vi "系统设置.vi"() -> ()   [LabVIEW 2016]
uses:
  <vilib>/Utility/miscctls.llb/LVPointTypeDef.ctl
  <vilib>/ptbypt/NI_PtbyPt.lvlib
  <vilib>/Utility/config.llb/NI_LVConfig.lvlib
  PLC/PLC.lvlib
panel:
  in  "模块启用配置":bool
  in  "短信报警设置":bool
  in  "首页显示设置":bool
  in  "跨度核查":bool
  in  "空白核查":bool
  out "选项卡控件":enum32{"自由设定", "国标协议", "流量设定"}(tab)
  in  "24H周期设置":bool[](xcontrol)
  in  "运行间隔":i16=4 min=1 max=24
  in  "流量阈值":dbl=4.0 min=1.0 max=24.0
  in  "时间阈值":u16=4 min=1 max=24
  in  "周期设置":enum16{"自由设定", "国标协议", "流量设定"}(ring)
  out "x = y?":bool
  in  "质控启动日期":string(combo)="关闭"
  in  "跨度核查时间":u16(ring)=6 items=["00H", "01H", "02H", "03H", "04H", "05H", "06H", "07H", "08H", "09H", "10H", "11H", "12H", "13H", "14H", "15H", "16H", "17H", "18H", "19H", "20H", "21H", "22H", "23H", "关闭"]
  in  "空白核查时间":u16(ring)=2 items=["00H", "01H", "02H", "03H", "04H", "05H", "06H", "07H", "08H", "09H", "10H", "11H", "12H", "13H", "14H", "15H", "16H", "17H", "18H", "19H", "20H", "21H", "22H", "23H", "关闭"]
  in  "CODCr":bool
  in  "总磷总氮":bool
  in  "氨氮":bool
  in  "CODmn":bool
  in  "多参数":bool
  in  "输入密码":dbl
  in  "布尔":bool
  in  "副屏显示设置":bool
  in  "开机启动":bool caption="氨氮禁用"
  in  "运行模式":enum16{"维护模式", "常规模式", "应急模式", "质控模式"}(ring)
  # "注：周期设置分为自由设定和国标协议两种。\n1：选择自由设定情况下：运行间隔将不可选用并变灰色，周期设置可自由手动勾选\n2：选择国标协议情况下：周期时间将由运行间隔选择的时间决定，下方周期设置被禁用并无法手动勾选。\n3：选择流量设定情况下：瞬时流量连续超过流量阈值到达时间阈值设定值，仪器将自动开启测量。"
  # "自动运行启动参数"
  # "质控频次："
  # "空白核查时间："
  # "跨度核查时间："
  # "启动周期设置"
  # "m3/S"
  # "秒"
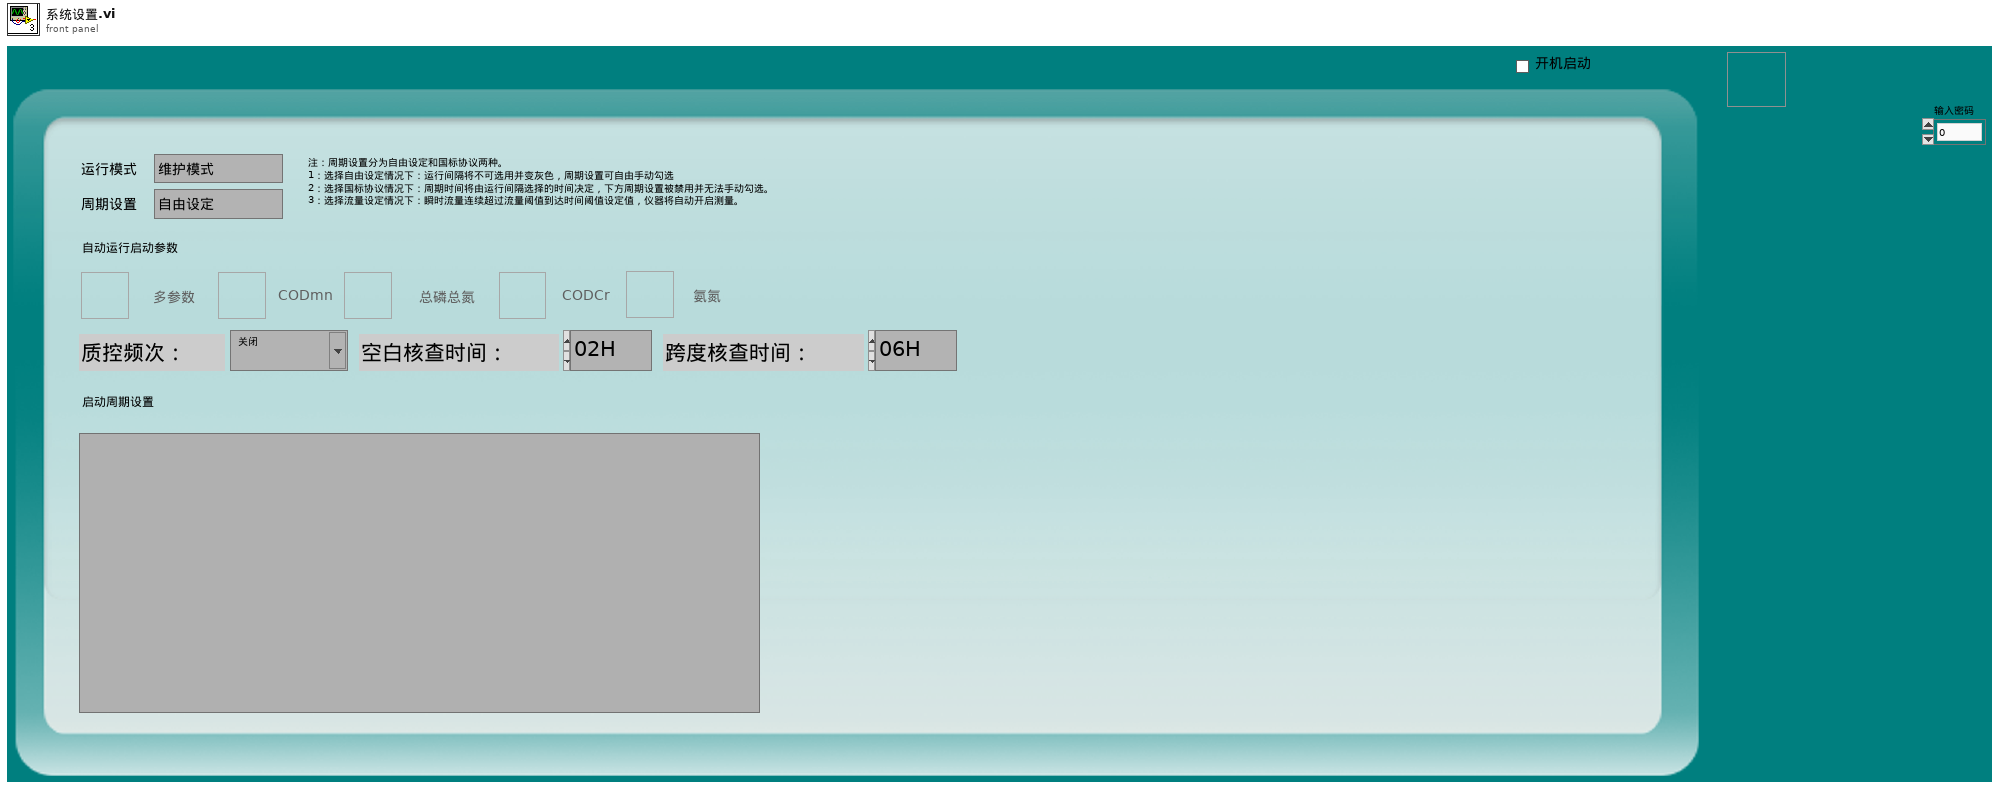
[diagram p1: front panel]
types:
  T1 = typedef "NI_LVConfig.lvlib/Config Data RefNum.ctl" = refnum<k1>
  T2 = typedef "LVPointTypeDef.ctl" = cluster{"Horizontal":i16, "Vertical":i16}
  T3 = enum8{"Enabled", "Disabled", "Disabled and Grayed Out"}
  T4 = enum32{"Bad", "Idle", "Run top level", "Running"}
  T5 = enum32{"Invalid", "Standard", "Closed", "Hidden", "Minimized", "Maximized"}
  T6 = cluster{"运行模式":enum16{"维护模式", "常规模式", "应急模式", "质控模式"}}
  T7 = cluster{"测量模式":enum16{"水样测量", "标样核查", "零点核查", "跨度核查", "空白测试", "加标回收", "平行样", "校零", "校标"}}
  T8 = cluster{"站号":u16, "量程切换":enum32{"H", "L", "AUTO"}, "控制命令":enum16{"启动测量", "标样核查", "零点核查", "跨度核查", "空白测试", "平行样测试", "加标回收", "空白校准", "标样校准", "初始化（清洗）", "停止测试", "仪器重启", "校时", "模式设置", "测量间隔设置"}, "模式设置":enum16{"待机", "连续模式", "周期模式", "定点模式", "受控模式", "手动模式"}, "测量间隔":u16}
  T9 = enum16{"启动测量", "标样核查", "零点核查", "跨度核查", "空白测试", "平行样测试", "加标回收", "空白校准", "标样校准", "初始化（清洗）", "停止测试", "仪器重启", "校时", "模式设置", "测量间隔设置"}
  T10 = cluster{"测试模式":enum16{"正常测试", "集成干预"}, "参数启用":cluster{"氨氮":bool, "总磷总氮":bool, "CODMn":bool, "CODcr":bool, "多参数":bool}}
  T11 = typedef "LVDateTimeRec.ctl" = cluster{"秒数的小数部分":dbl, "秒":i32, "分":i32, "时":i32, "日":i32, "月":i32, "年":i32, "天数（周）":i32, "天数（年）":i32, "DST":i32}
  T12 = cluster{"水样测试量程模式":enum16{"H", "L", "AUTO"}, "空白核查量程模式":enum16{"H", "L", "AUTO"}, "跨度核查量程模式":enum16{"H", "L", "AUTO"}}
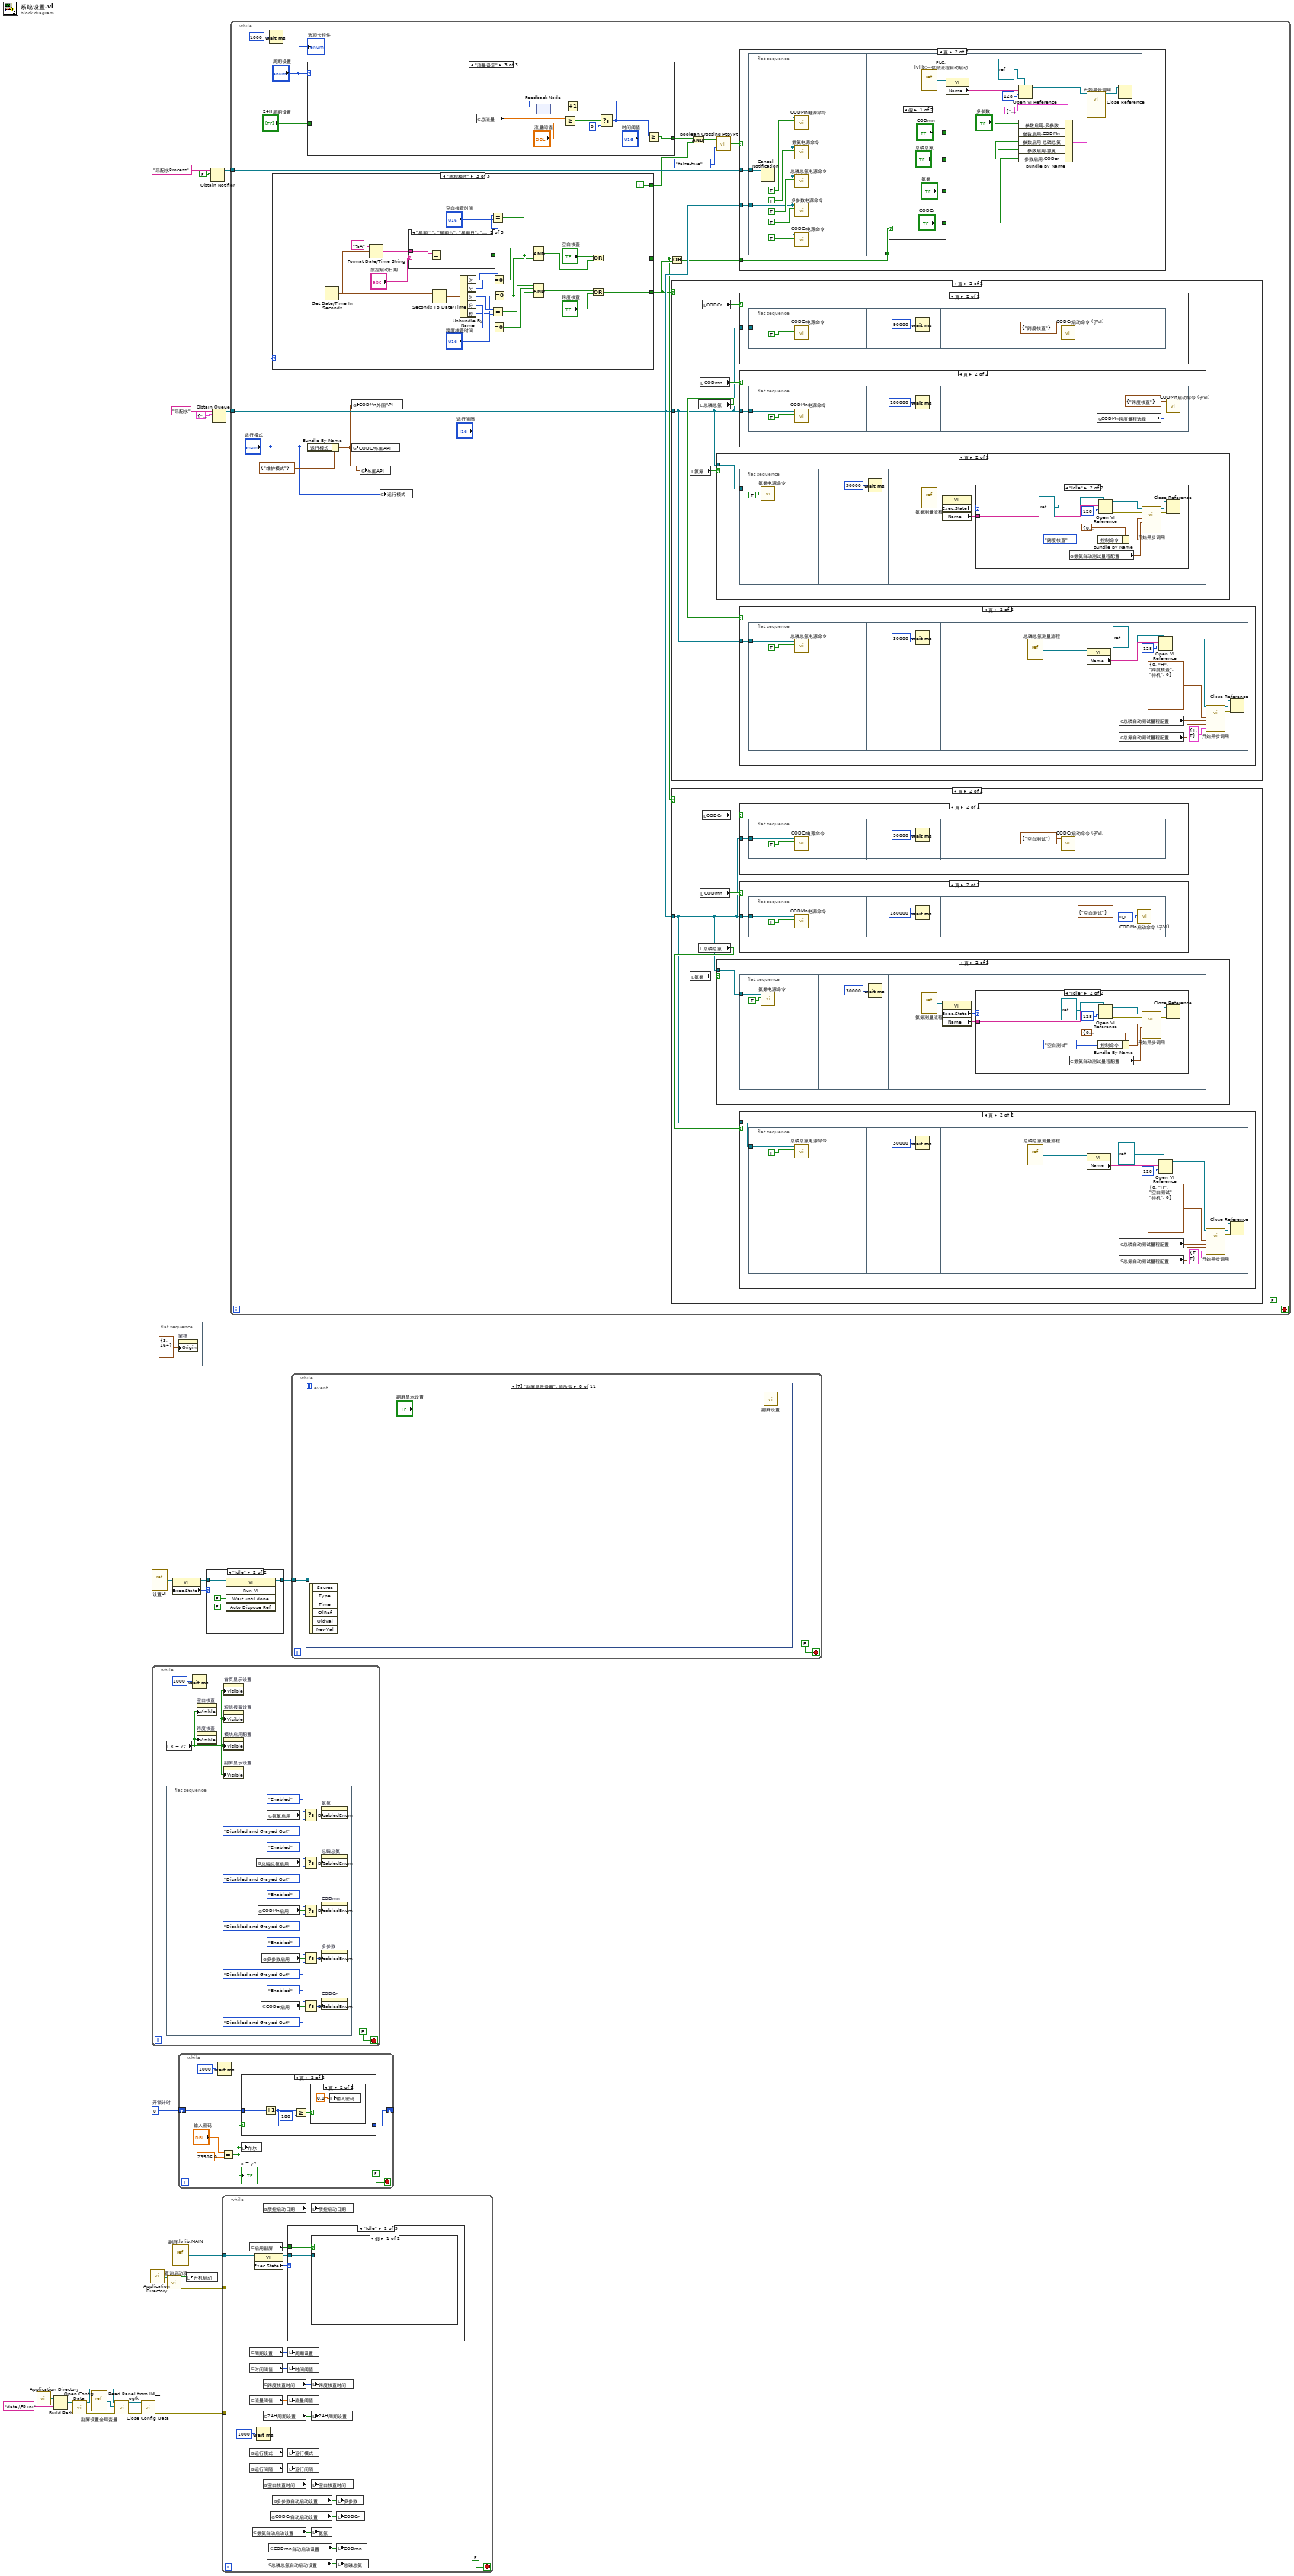
[diagram p0: block diagram]
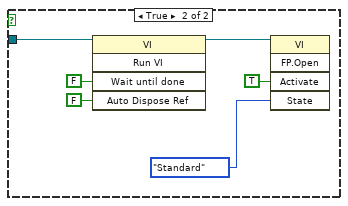
[diagram p6: hidden frame]
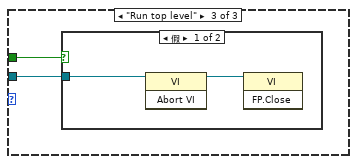
[diagram p7: hidden frame]
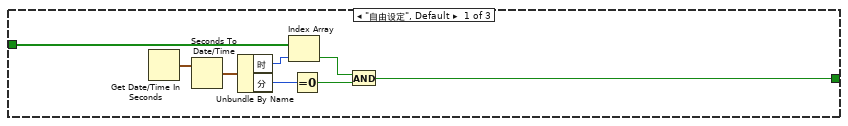
[diagram p9: hidden frame]
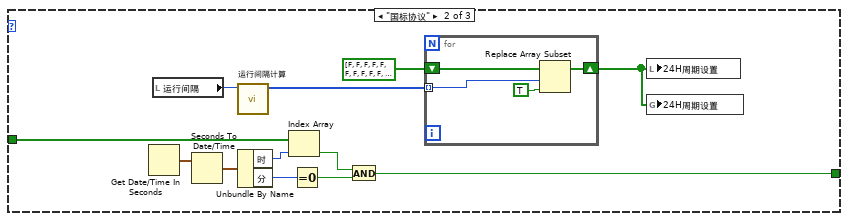
[diagram p10: hidden frame]
diagram:
  w19 = u32 0  # 开锁计时
  n1 = call <vilib>:"Application Directory.vi"() -> ("Application Directory"=w1:path)
  n2 = Build Path(base path=w1, name or relative path="data\\FP.ini" ("名称或相对路径")) -> (appended path=w8:path)
  n3 = call <vilib>:"Open Config Data.vi"("configuration file path"=w8) -> ("error out"=w7:errorcluster, "refnum"=w4:T1)  [unwired: 8 in, 1 out]
  n4 = vi-ref "副屏设置全局变量.vi"() -> (w5:refnum<vi>)
  n5 = call <userlib>:"Read Panel from INI__ogtk.vi"("error in (no error)"=w7, "VI ref"=w5, "refnum"=w4) -> ("error out"=w6:errorcluster, "refnum out"=w3:T1)  [unwired: 7 in]
  n6 = call <vilib>:"Close Config Data.vi"("error in (no error)"=w6, "refnum"=w3) -> ("error out"=w2:errorcluster)  [unwired: 8 in, 1 out]
  n7 = call <vilib>:"Application Directory.vi"() -> ("Application Directory"=w21:path)
  n8 = flat-sequence {
    frame #0 {
      n9 = property on="窗格" class="Pane"("Origin"=T2 {"Horizontal"=3, "Vertical"=164} ("原点")) -> ()  [unwired: 2 in, 2 out]
    }
  }
  n10 = vi-ref "设置UI.vi"() -> (w14:refnum<vi>)
  n11 = while {
    stop <- FALSE stop-if-true
    n12 = local read "x = y?"() -> (w26:bool)
    n13 = flat-sequence {
      frame #0 {
        n14 = global read "系统设置全局变量.vi" "总磷总氮启用"() -> (w36:bool)
        n15 = global read "系统设置全局变量.vi" "CODMn启用"() -> (w34:bool)
        n16 = global read "系统设置全局变量.vi" "CODcr启用"() -> (w35:bool)
        n17 = global read "系统设置全局变量.vi" "多参数启用"() -> (w33:bool)
        n18 = global read "系统设置全局变量.vi" "氨氮启用"() -> (w29:bool)
        n19 = Select(t=T3."Enabled" ("禁用"), s=w29, f=T3."Disabled and Grayed Out" ("禁用")) -> (s? t:f=w37:T3)
        n20 = Select(t=T3."Enabled" ("禁用"), s=w36, f=T3."Disabled and Grayed Out" ("禁用")) -> (s? t:f=w31:T3)
        n21 = Select(t=T3."Enabled" ("禁用"), s=w34, f=T3."Disabled and Grayed Out" ("禁用")) -> (s? t:f=w38:T3)
        n22 = Select(t=T3."Enabled" ("禁用"), s=w33, f=T3."Disabled and Grayed Out" ("禁用")) -> (s? t:f=w32:T3)
        n23 = Select(t=T3."Enabled" ("禁用"), s=w35, f=T3."Disabled and Grayed Out" ("禁用")) -> (s? t:f=w48:T3)
        n24 = property on="氨氮" class="Bool (严格)"("DisabledEnum"=w37) -> ()  [unwired: 2 in, 2 out]
        n25 = property on="总磷总氮" class="Bool (严格)"("DisabledEnum"=w31) -> ()  [unwired: 2 in, 2 out]
        n26 = property on="CODmn" class="Bool (严格)"("DisabledEnum"=w38) -> ()  [unwired: 2 in, 2 out]
        n27 = property on="多参数" class="Bool (严格)"("DisabledEnum"=w32) -> ()  [unwired: 2 in, 2 out]
        n28 = property on="CODCr" class="Bool (严格)"("DisabledEnum"=w48) -> ()  [unwired: 2 in, 2 out]
      }
    }
    n29 = Wait (ms)(milliseconds to wait=u32 1000 ("等待时间（毫秒）")) -> ()  [unwired: 1 out]
    n30 = property on="空白核查" class="Bool"("Visible"=w26) -> ()  [unwired: 2 in, 2 out]
    n31 = property on="跨度核查" class="Bool"("Visible"=w26) -> ()  [unwired: 2 in, 2 out]
    n32 = property on="首页显示设置" class="Bool"("Visible"=w26) -> ()  [unwired: 2 in, 2 out]
    n33 = property on="短信报警设置" class="Bool"("Visible"=w26) -> ()  [unwired: 2 in, 2 out]
    n34 = property on="模块启用配置" class="Bool"("Visible"=w26) -> ()  [unwired: 2 in, 2 out]
    n35 = property on="副屏显示设置" class="Bool"("Visible"=w26) -> ()  [unwired: 2 in, 2 out]
  }
  n36 = call "查询启动项.vi"("启动文件路径"=w21) -> ("error out"=w10:errorcluster, "包含启动项"=w20:bool)  [unwired: 9 in]
  n37 = property class="VI"(reference=w14) -> (reference out=w12:refnum<vi>, "Exec.State"=w13:T4)  [unwired: 1 in, 1 out]
  n38 = vi-ref "副屏.lvlib:MAIN.vi"() -> (w15:refnum<vi>)
  n39 = while {
    shift-right: [w50] -> _
    shift-left: w19 -> [w51]
    stop <- FALSE stop-if-true
    n40 = Wait (ms)(milliseconds to wait=u32 1000 ("等待时间（毫秒）")) -> ()  [unwired: 1 out]
    n41 = Equal?(x="输入密码", y=23506.0) -> (x = y?=w49:bool)
    "x = y?" <- w49
    n42 = case shown="真" w49 {
      tunnel: w51 -> [_ w59]
      tunnel: [_ w58] -> w50
      frame False {
      }
      frame True {
        n43 = Increment(x=w59) -> (x+1=w58:u32)
        n44 = Greater Or Equal?(x=w58, y=u32 180) -> (x >= y?=w56:bool)
        n45 = case shown="真" w56 {
          frame False {
          }
          frame True {
            n46 = local write "输入密码"(0.0 ("输入密码")) -> ()
          }
        }
      }
    }
    n47 = local write "布尔"(w49) -> ()
  }
  n48 = local write "开机启动"(w20) -> ()
  n49 = case shown="\"Idle\"" w13 {
    tunnel: w12 -> [w61 w65]
    tunnel: [w61 w64] -> w11
    frame "Bad", Default {
    }
    frame "Idle" {
      n50 = invoke class="VI" method="Run VI"(reference=w65, "Wait until done"=FALSE ("结束前等待"), "Auto Dispose Ref"=FALSE ("自动销毁引用")) -> (reference out=w64:refnum<vi>)  [unwired: 2 in, 4 out]
    }
  }
  n51 = Obtain Notifier(name (unnamed)="采配水Process" ("名称（未命名）"), notification data type=FALSE) -> (notifier out=w22:refnum<notifier>)  [unwired: 2 in, 2 out]
  n52 = Obtain Queue(name (unnamed)="采配水" ("名称（未命名）"), element data type=cluster{"命令":string, "数据":variant} {"命令"="", "数据"=variant}) -> (queue out=w16:refnum<queue>)  [unwired: 3 in, 2 out]
  n53 = while {
    tunnel: w15 -> [w77]
    tunnel: w10 -> [_]
    tunnel: w2 -> [_]
    stop <- FALSE stop-if-true
    n54 = global read "副屏设置全局变量.vi" "启用副屏"() -> (w75:bool)
    n55 = global read "系统设置全局变量.vi" "周期设置"() -> (w70:enum16{"自由设定", "国标协议", "流量设定"})
    n56 = global read "系统设置全局变量.vi" "时间阈值"() -> (w66:u16)
    n57 = global read "系统设置全局变量.vi" "流量阈值"() -> (w67:dbl)
    n58 = global read "系统设置全局变量.vi" "运行模式"() -> (w68:enum16{"维护模式", "常规模式", "应急模式", "质控模式"})
    n59 = global read "系统设置全局变量.vi" "运行间隔"() -> (w69:i16)
    n60 = global read "系统设置全局变量.vi" "氨氮自动启动设置"() -> (w82:bool)
    n61 = property class="VI"(reference=w77) -> (reference out=w74:refnum<vi>, "Exec.State"=w76:T4)  [unwired: 1 in, 1 out]
    n62 = Wait (ms)(milliseconds to wait=u32 1000 ("等待时间（毫秒）")) -> ()  [unwired: 1 out]
    n63 = global read "系统设置全局变量.vi" "质控启动日期"() -> (w73:string)
    n64 = global read "系统设置全局变量.vi" "跨度核查时间"() -> (w71:u16)
    n65 = global read "系统设置全局变量.vi" "24H周期设置"() -> (w83:bool[])
    n66 = global read "系统设置全局变量.vi" "空白核查时间"() -> (w72:u16)
    n67 = global read "系统设置全局变量.vi" "总磷总氮自动启动设置"() -> (w80:bool)
    n68 = global read "系统设置全局变量.vi" "CODmn自动启动设置"() -> (w79:bool)
    n69 = global read "系统设置全局变量.vi" "CODCr自动启动设置"() -> (w81:bool)
    n70 = global read "系统设置全局变量.vi" "多参数自动启动设置"() -> (w78:bool)
    n71 = case shown="\"Idle\"" w76 {
      tunnel: w75 -> [_ w86 w94]
      tunnel: w74 -> [_ w87 w95]
      frame "Bad", Default {
      }
      frame "Idle" {
        n72 = case shown="假" w86 {
          tunnel: w87 -> [_ w93]
          frame False {
          }
          frame True {
            n73 = invoke class="VI" method="Run VI"(reference=w93, "Wait until done"=FALSE ("结束前等待"), "Auto Dispose Ref"=FALSE ("自动销毁引用")) -> (reference out=w88:refnum<vi>)  [unwired: 2 in, 4 out]
            n74 = invoke class="VI" method="FP.Open"(reference=w88, "Activate"=TRUE ("激活？"), "State"=T5."Standard" ("状态")) -> ()  [unwired: 2 in, 5 out]
          }
        }
      }
      frame "Run top level" {
        n75 = case shown="假" w94 {
          tunnel: w95 -> [w96 _]
          frame False {
            n76 = invoke class="VI" method="Abort VI"(reference=w96) -> (reference out=w97:refnum<vi>)  [unwired: 2 in, 2 out]
            n77 = invoke class="VI" method="FP.Close"(reference=w97) -> ()  [unwired: 2 in, 3 out]
          }
          frame True {
          }
        }
      }
    }
    n78 = local write "周期设置"(w70) -> ()
    n79 = local write "时间阈值"(w66) -> ()
    n80 = local write "流量阈值"(w67) -> ()
    n81 = local write "运行模式"(w68) -> ()
    n82 = local write "运行间隔"(w69) -> ()
    n83 = local write "质控启动日期"(w73) -> ()
    n84 = local write "跨度核查时间"(w71) -> ()
    n85 = local write "24H周期设置"(w83) -> ()
    n86 = local write "空白核查时间"(w72) -> ()
    n87 = local write "氨氮"(w82) -> ()
    n88 = local write "多参数"(w78) -> ()
    n89 = local write "CODCr"(w81) -> ()
    n90 = local write "CODmn"(w79) -> ()
    n91 = local write "总磷总氮"(w80) -> ()
  }
  n92 = while {
    tunnel: w22 -> [w112]
    tunnel: w16 -> [w108]
    stop <- FALSE stop-if-true
    n93 = Wait (ms)(milliseconds to wait=u32 1000 ("等待时间（毫秒）")) -> ()  [unwired: 1 out]
    n94 = case shown="\"质控模式\"" "运行模式" {
      tunnel: [_ _ w276] -> w102
      tunnel: [_ _ w280] -> w101
      tunnel: [_ TRUE TRUE] -> w105
      frame "维护模式", Default {
      }
      frame "常规模式" {
      }
      frame "质控模式" {
        n95 = Get Date/Time In Seconds() -> (seconds since 1Jan1904=w287:timestamp)
        n96 = Format Date/Time String(time format string (%c)="%A" ("时间格式字符串(%c)"), seconds (now)=w287) -> (date/time string=w285:string)  [unwired: 1 in]
        n97 = case shown="\"星期二\", \"星期六\", \"星期日\", \"星期三\", \"星期四\", \"星期五\", \"星期一\"" "质控启动日期" {
          selector: "质控启动日期" -> [w303 _ _]
          tunnel: [w302 TRUE FALSE] -> w288
          tunnel: w285 -> [w301 _ _]
          frame "星期二", "星期六", "星期日", "星期三", "星期四", "星期五", "星期一" {
            n98 = Equal?(x=w301, y=w303) -> (x = y?=w302:bool)
          }
          frame "每天" {
          }
          frame "关闭", Default {
          }
        }
        n99 = Seconds To Date/Time(time stamp (now)=w287) -> (date time rec=w300:T11)  [unwired: 1 in]
        n100 = Unbundle By Name(w300) -> ("时"=w299:i32, "分"=w297:i32, "时"=w293:i32, "分"=w292:i32, "秒"=w284:i32)
        n101 = Equal?(x=w299, y="空白核查时间") -> (x = y?=w296:bool)
        n102 = Equal?(x=w293, y="跨度核查时间") -> (x = y?=w291:bool)
        n103 = Equal To 0?(x=w297) -> (x = 0?=w295:bool)
        n104 = Equal To 0?(x=w292) -> (x = 0?=w290:bool)
        n105 = Equal To 0?(x=w284) -> (x = 0?=w283:bool)
        n106 = Compound Arithmetic op=AND ("复合运算")(w295, w296, w288, w283) -> (w281:bool)
        n107 = Compound Arithmetic op=AND ("复合运算")(w291, w290, w288, w283) -> (w278:bool)
        n108 = Or(x="空白核查", y=w281) -> (x .or. y?=w280:bool)
        n109 = Or(x=w278, y="跨度核查") -> (x .or. y?=w276:bool)
      }
    }
    n110 = case shown="\"流量设定\"" "周期设置" {
      tunnel: [w116 w123 w139] -> w104
      tunnel: "24H周期设置" -> [w115 w124 _]
      frame "自由设定", Default {
        n111 = Get Date/Time In Seconds() -> (seconds since 1Jan1904=w117:timestamp)
        n112 = Seconds To Date/Time(time stamp (now)=w117) -> (date time rec=w118:T11)  [unwired: 1 in]
        n113 = Unbundle By Name(w118) -> ("时"=w121:i32, "分"=w119:i32)
        n114 = Index Array(array=w115, index=w121) -> (element=w122:bool)
        n115 = Equal To 0?(x=w119) -> (x = 0?=w120:bool)
        n116 = And(x=w122, y=w120) -> (x .and. y?=w116:bool)
      }
      frame "国标协议" {
        n117 = Get Date/Time In Seconds() -> (seconds since 1Jan1904=w125:timestamp)
        n118 = local read "运行间隔"() -> (w134:i16)
        n119 = Seconds To Date/Time(time stamp (now)=w125) -> (date time rec=w126:T11)  [unwired: 1 in]
        n120 = call "运行间隔计算.vi"("运行周期"=w134) -> ("数组"=w133:i32[])  [unwired: 10 in]
        n121 = Unbundle By Name(w126) -> ("时"=w129:i32, "分"=w127:i32)
        n122 = Index Array(array=w124, index=w129) -> (element=w130:bool)
        n123 = Equal To 0?(x=w127) -> (x = 0?=w128:bool)
        n124 = And(x=w130, y=w128) -> (x .and. y?=w123:bool)
        n125 = for {
          tunnel: w133 -> [w137] mode=indexing
          shift-right: [w135] -> w131
          shift-left: bool[] [FALSE, FALSE, FALSE, FALSE, FALSE, FALSE, FALSE, FALSE, FALSE, FALSE, FALSE, FALSE, FALSE, FALSE, FALSE, FALSE, FALSE, FALSE, FALSE, FALSE, FALSE, FALSE, FALSE, FALSE] ("24H周期设置") -> [w138]
          n126 = Replace Array Subset(array=w138, new element=TRUE ("新元素/子数组"), index=w137) -> (w135:bool[])
        }
        n127 = local write "24H周期设置"(w131) -> ()
        n128 = global write "系统设置全局变量.vi" "24H周期设置"(w131) -> ()
      }
      frame "流量设定" {
        n129 = global read "流量计全局变量.vi" "总流量"() -> (w147:dbl)
        n130 = feedback #1() -> (w144:i16)  [unwired: 1 in]
        n131 = Greater Or Equal?(x=w147, y="流量阈值") -> (x >= y?=w142:bool)
        n132 = Increment(x=w144) -> (x+1=w143:i16)
        n133 = Select(t=w143, s=w142, f=i16 0) -> (s? t:f=w141:i16)
        n134 = feedback-in #1(w141) -> ()
        n135 = Greater Or Equal?(x=w141, y="时间阈值") -> (x >= y?=w139:bool)
      }
    }
    n136 = Bundle By Name(cluster=T6 {"运行模式"=enum."维护模式"} ("外围API"), "运行模式"="运行模式") -> (w99:T6)
    n137 = global write "CODMN外部API.vi" "CODMn外围API"(w99) -> ()
    n138 = global write "CODCr外部API.vi" "CODCr外围API"(w99) -> ()
    n139 = global write "VAR氨氮全局变量.vi" "外围API"(w99) -> ()
    n140 = global write "多参数全局变量.vi" "运行模式"("运行模式") -> ()
    n141 = Or(x=w101, y=w102) -> (x .or. y?=w100:bool)
    n142 = case shown="真" w102 {
      tunnel: w108 -> [_ w148]
      frame False {
      }
      frame True {
        n143 = local read "氨氮"() -> (w152:bool)
        n144 = local read "总磷总氮"() -> (w151:bool)
        n145 = local read "CODmn"() -> (w150:bool)
        n146 = local read "CODCr"() -> (w149:bool)
        n147 = case shown="真" w152 {
          tunnel: w148 -> [_ w179]
          frame False {
          }
          frame True {
            n148 = flat-sequence {
              tunnel: w179 -> [w180]
              frame #0 {
                n149 = call "氨氮电源命令.vi"("通电/断电"=TRUE, "队列"=w180) -> ()  [unwired: 9 in, 1 out]
              }
              frame #1 {
                n150 = Wait (ms)(milliseconds to wait=u32 30000 ("等待时间（毫秒）")) -> ()  [unwired: 1 out]
              }
              frame #2 {
                n151 = vi-ref "氨氮测量流程.vi"() -> (w185:refnum<vi>)
                n152 = property class="VI"(reference=w185) -> ("Exec.State"=w183:T4, "Name"=w184:string)  [unwired: 1 in, 2 out]
                n153 = case shown="\"Idle\"" w183 {
                  tunnel: w184 -> [_ w193]
                  frame "Bad", Default {
                  }
                  frame "Idle" {
                    n154 = global read "氨氮断电保存全局变量.vi" "氨氮自动测试量程配置"() -> (w187:T12)
                    n155 = Bundle By Name(cluster=T8 {"站号"=0, "量程切换"=enum."H", "控制命令"=enum."启动测量", "模式设置"=enum."待机", "测量间隔"=0} ("参数"), "控制命令"=T9."跨度核查") -> (w188:T8)
                    n156 = Open VI Reference(type specifier VI Refnum (for type only)=refnum<vi> refnum, vi path=w193, options=128 ("选项")) -> (vi reference=w189:refnum<vi>, error out=w194:errorcluster)  [unwired: 3 in]
                    n157 = call-by-ref "开始异步调用"(reference=w189, error in=w194, "量程模式"=w187, "参数"=w188) -> (reference out=w195:refnum<vi>, error out=w196:errorcluster)  [unwired: 10 in]
                    n158 = Close Reference(reference=w195, error in (no error)=w196) -> ()  [unwired: 1 out]
                  }
                }
              }
            }
          }
        }
        n159 = case shown="真" w149 {
          tunnel: w148 -> [_ w153]
          frame False {
          }
          frame True {
            n160 = flat-sequence {
              tunnel: w153 -> [w154]
              frame #0 {
                n161 = call "CODCr电源命令.vi"("通电/断电"=TRUE, "队列"=w154) -> ()  [unwired: 9 in, 1 out]
              }
              frame #1 {
                n162 = Wait (ms)(milliseconds to wait=u32 90000 ("等待时间（毫秒）")) -> ()  [unwired: 1 out]
              }
              frame #2 {
                n163 = call "CODCr启动命令 (子VI).vi"("启动测量模式"=T7 {"测量模式"=enum."跨度核查"}) -> ()  [unwired: 11 in]
              }
            }
          }
        }
        n164 = case shown="真" w150 {
          tunnel: w148 -> [_ w158]
          frame False {
          }
          frame True {
            n165 = flat-sequence {
              tunnel: w158 -> [w159]
              frame #0 {
                n166 = call "CODMn电源命令.vi"("通电/断电"=TRUE, "队列"=w159) -> ()  [unwired: 9 in, 1 out]
              }
              frame #1 {
                n167 = Wait (ms)(milliseconds to wait=u32 180000 ("等待时间（毫秒）")) -> ()  [unwired: 1 out]
              }
              frame #2 {
              }
              frame #3 {
                n168 = global read "CODMn断电保存全局变量.vi" "CODMn跨度量程选择"() -> (w162:enum32{"H", "L", "AUTO"})
                n169 = call "CODMn启动命令 (子VI).vi"("CODMn量程切换"=w162, "启动测量模式"=T7 {"测量模式"=enum."跨度核查"}) -> ()  [unwired: 10 in]
              }
            }
          }
        }
        n170 = case shown="真" w151 {
          tunnel: w148 -> [_ w164]
          frame False {
          }
          frame True {
            n171 = flat-sequence {
              tunnel: w164 -> [w166]
              frame #0 {
                n172 = call "总磷总氮电源命令.vi"("通电/断电"=TRUE, "队列"=w166) -> ()  [unwired: 9 in, 1 out]
              }
              frame #1 {
                n173 = Wait (ms)(milliseconds to wait=u32 30000 ("等待时间（毫秒）")) -> ()  [unwired: 1 out]
              }
              frame #2 {
                n174 = vi-ref "总磷总氮测量流程.vi"() -> (w176:refnum<vi>)
                n175 = property class="VI"(reference=w176) -> ("Name"=w177:string)  [unwired: 1 in, 2 out]
                n176 = global read "总磷总氮断电保存全局变量.vi" "总磷自动测试量程配置"() -> (w171:T12)
                n177 = global read "总磷总氮断电保存全局变量.vi" "总氮自动测试量程配置"() -> (w170:T12)
                n178 = Open VI Reference(type specifier VI Refnum (for type only)=refnum<vi> refnum, vi path=w177, options=128 ("选项")) -> (vi reference=w175:refnum<vi>)  [unwired: 3 in, 1 out]
                n179 = call-by-ref "开始异步调用"(reference=w175, "启动参数"=cluster{"总磷":bool, "总氮":bool} {"总磷"=TRUE, "总氮"=TRUE}, "总氮量程模式"=w170, "总磷量程模式"=w171, "参数"=T8 {"站号"=0, "量程切换"=enum."H", "控制命令"=enum."跨度核查", "模式设置"=enum."待机", "测量间隔"=0}) -> (reference out=w174:refnum<vi>, error out=w173:errorcluster)  [unwired: 9 in]
                n180 = Close Reference(reference=w174, error in (no error)=w173) -> ()  [unwired: 1 out]
              }
            }
          }
        }
      }
    }
    n181 = case shown="真" w101 {
      tunnel: w108 -> [_ w197]
      frame False {
      }
      frame True {
        n182 = local read "氨氮"() -> (w201:bool)
        n183 = local read "总磷总氮"() -> (w200:bool)
        n184 = local read "CODmn"() -> (w199:bool)
        n185 = local read "CODCr"() -> (w198:bool)
        n186 = case shown="真" w201 {
          tunnel: w197 -> [_ w228]
          frame False {
          }
          frame True {
            n187 = flat-sequence {
              tunnel: w228 -> [w229]
              frame #0 {
                n188 = call "氨氮电源命令.vi"("通电/断电"=TRUE, "队列"=w229) -> ()  [unwired: 9 in, 1 out]
              }
              frame #1 {
                n189 = Wait (ms)(milliseconds to wait=u32 30000 ("等待时间（毫秒）")) -> ()  [unwired: 1 out]
              }
              frame #2 {
                n190 = vi-ref "氨氮测量流程.vi"() -> (w234:refnum<vi>)
                n191 = property class="VI"(reference=w234) -> ("Exec.State"=w232:T4, "Name"=w233:string)  [unwired: 1 in, 2 out]
                n192 = case shown="\"Idle\"" w232 {
                  tunnel: w233 -> [_ w242]
                  frame "Bad", Default {
                  }
                  frame "Idle" {
                    n193 = global read "氨氮断电保存全局变量.vi" "氨氮自动测试量程配置"() -> (w235:T12)
                    n194 = Bundle By Name(cluster=T8 {"站号"=0, "量程切换"=enum."H", "控制命令"=enum."启动测量", "模式设置"=enum."待机", "测量间隔"=0} ("参数"), "控制命令"=T9."空白测试") -> (w237:T8)
                    n195 = Open VI Reference(type specifier VI Refnum (for type only)=refnum<vi> refnum, vi path=w242, options=128 ("选项")) -> (vi reference=w238:refnum<vi>, error out=w243:errorcluster)  [unwired: 3 in]
                    n196 = call-by-ref "开始异步调用"(reference=w238, error in=w243, "量程模式"=w235, "参数"=w237) -> (reference out=w244:refnum<vi>, error out=w245:errorcluster)  [unwired: 10 in]
                    n197 = Close Reference(reference=w244, error in (no error)=w245) -> ()  [unwired: 1 out]
                  }
                }
              }
            }
          }
        }
        n198 = case shown="真" w198 {
          tunnel: w197 -> [_ w202]
          frame False {
          }
          frame True {
            n199 = flat-sequence {
              tunnel: w202 -> [w203]
              frame #0 {
                n200 = call "CODCr电源命令.vi"("通电/断电"=TRUE, "队列"=w203) -> ()  [unwired: 9 in, 1 out]
              }
              frame #1 {
                n201 = Wait (ms)(milliseconds to wait=u32 90000 ("等待时间（毫秒）")) -> ()  [unwired: 1 out]
              }
              frame #2 {
                n202 = call "CODCr启动命令 (子VI).vi"("启动测量模式"=T7 {"测量模式"=enum."空白测试"}) -> ()  [unwired: 11 in]
              }
            }
          }
        }
        n203 = case shown="真" w199 {
          tunnel: w197 -> [_ w207]
          frame False {
          }
          frame True {
            n204 = flat-sequence {
              tunnel: w207 -> [w208]
              frame #0 {
                n205 = call "CODMn电源命令.vi"("通电/断电"=TRUE, "队列"=w208) -> ()  [unwired: 9 in, 1 out]
              }
              frame #1 {
                n206 = Wait (ms)(milliseconds to wait=u32 180000 ("等待时间（毫秒）")) -> ()  [unwired: 1 out]
              }
              frame #2 {
              }
              frame #3 {
                n207 = call "CODMn启动命令 (子VI).vi"("CODMn量程切换"=enum32{"H", "L", "AUTO"}."L", "启动测量模式"=T7 {"测量模式"=enum."空白测试"}) -> ()  [unwired: 10 in]
              }
            }
          }
        }
        n208 = case shown="真" w200 {
          tunnel: w197 -> [_ w213]
          frame False {
          }
          frame True {
            n209 = flat-sequence {
              tunnel: w213 -> [w215]
              frame #0 {
                n210 = call "总磷总氮电源命令.vi"("通电/断电"=TRUE, "队列"=w215) -> ()  [unwired: 9 in, 1 out]
              }
              frame #1 {
                n211 = Wait (ms)(milliseconds to wait=u32 30000 ("等待时间（毫秒）")) -> ()  [unwired: 1 out]
              }
              frame #2 {
                n212 = vi-ref "总磷总氮测量流程.vi"() -> (w225:refnum<vi>)
                n213 = property class="VI"(reference=w225) -> ("Name"=w226:string)  [unwired: 1 in, 2 out]
                n214 = global read "总磷总氮断电保存全局变量.vi" "总磷自动测试量程配置"() -> (w219:T12)
                n215 = global read "总磷总氮断电保存全局变量.vi" "总氮自动测试量程配置"() -> (w218:T12)
                n216 = Open VI Reference(type specifier VI Refnum (for type only)=refnum<vi> refnum, vi path=w226, options=128 ("选项")) -> (vi reference=w224:refnum<vi>)  [unwired: 3 in, 1 out]
                n217 = call-by-ref "开始异步调用"(reference=w224, "启动参数"=cluster{"总磷":bool, "总氮":bool} {"总磷"=TRUE, "总氮"=TRUE}, "总氮量程模式"=w218, "总磷量程模式"=w219, "参数"=T8 {"站号"=0, "量程切换"=enum."H", "控制命令"=enum."空白测试", "模式设置"=enum."待机", "测量间隔"=0}) -> (reference out=w223:refnum<vi>, error out=w222:errorcluster)  [unwired: 9 in]
                n218 = Close Reference(reference=w223, error in (no error)=w222) -> ()  [unwired: 1 out]
              }
            }
          }
        }
      }
    }
    n219 = And(x=w104, y=w105) -> (x .and. y?=w103:bool)
    n220 = call <vilib>:"Boolean Crossing PtByPt.vi"("direction"=enum16{"either", "false-true", "true-false"}."false-true", "input"=w103) -> ("crossing"=w110:bool)  [unwired: 1 in]
    n221 = case shown="真" w110 {
      tunnel: w112 -> [_ w248]
      tunnel: w108 -> [_ w247]
      tunnel: w100 -> [_ w246]
      frame False {
      }
      frame True {
        n222 = flat-sequence {
          tunnel: w248 -> [w255]
          tunnel: w247 -> [w249]
          tunnel: w246 -> [w259]
          frame #0 {
            n223 = Cancel Notification(0:w255) -> ()  [unwired: 1 in, 3 out]
            n224 = call "CODMn电源命令.vi"("通电/断电"=TRUE, "队列"=w249) -> ()  [unwired: 9 in, 1 out]
            n225 = call "氨氮电源命令.vi"("通电/断电"=TRUE, "队列"=w249) -> ()  [unwired: 9 in, 1 out]
            n226 = call "总磷总氮电源命令.vi"("通电/断电"=TRUE, "队列"=w249) -> ()  [unwired: 9 in, 1 out]
            n227 = call "多参数电源命令.vi"("通电/断电"=TRUE, "队列"=w249) -> ()  [unwired: 9 in, 1 out]
            n228 = call "CODCr电源命令.vi"("通电/断电"=TRUE, "队列"=w249) -> ()  [unwired: 9 in, 1 out]
          }
          frame #1 {
            n229 = case shown="假" w259 {
              tunnel: ["CODmn" _] -> w269
              tunnel: ["总磷总氮" _] -> w268
              tunnel: ["CODCr" _] -> w267
              tunnel: ["氨氮" _] -> w266
              frame False {
              }
              frame True {
              }
            }
            n230 = vi-ref "PLC.lvlib:一体站流程自动启动.vi"() -> (w263:refnum<vi>)
            n231 = property class="VI"(reference=w263) -> ("Name"=w264:string)  [unwired: 1 in, 2 out]
            n232 = Bundle By Name(cluster=T10 {"测试模式"=enum."正常测试", "参数启用"={"氨氮"=FALSE, "总磷总氮"=FALSE, "CODMn"=FALSE, "CODcr"=FALSE, "多参数"=FALSE}} ("参数"), "参数启用.多参数"="多参数", "参数启用.CODMn"=w269, "参数启用.总磷总氮"=w268, "参数启用.氨氮"=w266, "参数启用.CODcr"=w267) -> (w256:T10)
            n233 = Open VI Reference(type specifier VI Refnum (for type only)=refnum<vi> refnum, vi path=w264, options=128 ("选项")) -> (vi reference=w262:refnum<vi>)  [unwired: 3 in, 1 out]
            n234 = call-by-ref "开始异步调用"(reference=w262, "参数"=w256) -> (reference out=w261:refnum<vi>, error out=w260:errorcluster)  [unwired: 12 in]
            n235 = Close Reference(reference=w261, error in (no error)=w260) -> ()  [unwired: 1 out]
          }
        }
      }
    }
    "选项卡控件" <- "周期设置"
  }
  n236 = while {
    tunnel: w11 -> [w306]
    stop <- FALSE stop-if-true
    n237 = event shown="[7] \"副屏显示设置\": 值改变" {
      selector: _ -> [_ _ _ _ _ _ _ _ _ _ _]
      dyn-events: _ -> [_ _ _ _ _ _ _ _ _ _ _]
      timeout: _ -> [_ _ _ _ _ _ _ _ _ _ _]
      tunnel: w306 -> [_ _ _ _ _ _ _ _ _ w360 _]
      event Timeout {
        n238 = event-data() -> ()  [unwired: 1 in, 3 out]
      }
      event "模块启用配置": Value Change {
        n239 = event-data() -> ()  [unwired: 1 in, 6 out]
        n240 = call "模块启用配置框.vi"() -> ()  [unwired: 12 in]
      }
      event "24H周期设置", "运行模式", "多参数", "CODmn", "氨氮", "总磷总氮", "CODCr", "质控启动日期", "空白核查时间", "跨度核查时间", "运行间隔", "周期设置", "流量阈值", "时间阈值": Value Change {
        n241 = event-data() -> ()  [unwired: 1 in, 6 out]
        n242 = flat-sequence {
          frame #0 {
            n243 = local read "氨氮"() -> (w320:bool)
            n244 = local read "运行间隔"() -> (w311:i16)
            n245 = local read "流量阈值"() -> (w308:dbl)
            n246 = local read "总磷总氮"() -> (w318:bool)
            n247 = local read "周期设置"() -> (w310:enum16{"自由设定", "国标协议", "流量设定"})
            n248 = local read "时间阈值"() -> (w309:u16)
            n249 = local read "运行模式"() -> (w321:enum16{"维护模式", "常规模式", "应急模式", "质控模式"})
            n250 = local read "CODmn"() -> (w317:bool)
            n251 = local read "CODCr"() -> (w319:bool)
            n252 = local read "多参数"() -> (w316:bool)
            n253 = local read "空白核查时间"() -> (w313:u16)
            n254 = local read "质控启动日期"() -> (w314:string)
            n255 = local read "24H周期设置"() -> (w315:bool[])
            n256 = local read "跨度核查时间"() -> (w312:u16)
            n257 = global write "系统设置全局变量.vi" "氨氮自动启动设置"(w320) -> ()
            n258 = global write "系统设置全局变量.vi" "运行间隔"(w311) -> ()
            n259 = global write "系统设置全局变量.vi" "流量阈值"(w308) -> ()
            n260 = global write "系统设置全局变量.vi" "CODCr自动启动设置"(w319) -> ()
            n261 = global write "系统设置全局变量.vi" "总磷总氮自动启动设置"(w318) -> ()
            n262 = global write "系统设置全局变量.vi" "周期设置"(w310) -> ()
            n263 = global write "系统设置全局变量.vi" "CODmn自动启动设置"(w317) -> ()
            n264 = global write "系统设置全局变量.vi" "时间阈值"(w309) -> ()
            n265 = global write "系统设置全局变量.vi" "多参数自动启动设置"(w316) -> ()
            n266 = global write "系统设置全局变量.vi" "运行模式"(w321) -> ()
            n267 = global write "系统设置全局变量.vi" "空白核查时间"(w313) -> ()
            n268 = global write "系统设置全局变量.vi" "质控启动日期"(w314) -> ()
            n269 = global write "系统设置全局变量.vi" "24H周期设置"(w315) -> ()
            n270 = global write "系统设置全局变量.vi" "跨度核查时间"(w312) -> ()
          }
          frame #1 {
            n271 = call <vilib>:"Application Directory.vi"() -> ("Application Directory"=w335:path)
            n272 = Build Path(base path=w335, name or relative path="data\\sys.ini" ("名称或相对路径")) -> (appended path=w333:path)
            n273 = call <vilib>:"Open Config Data.vi"("configuration file path"=w333) -> ("error out"=w329:errorcluster, "refnum"=w332:T1)  [unwired: 8 in, 1 out]
            n274 = vi-ref "系统设置全局变量.vi"() -> (w331:refnum<vi>)
            n275 = call <userlib>:"Write Panel to INI__ogtk.vi"("error in (no error)"=w329, "VI ref"=w331, "refnum"=w332) -> ("error out"=w328:errorcluster, "refnum out"=w330:T1)  [unwired: 7 in]
            n276 = call <vilib>:"Close Config Data.vi"("error in (no error)"=w328, "refnum"=w330) -> ("error out"=w323:errorcluster, "file path"=w322:path)  [unwired: 8 in]
            n277 = Open/Create/Replace File(file path (use dialog)=w322, error in=w323) -> (refnum out=w326:refnum<file>, error out=w327:errorcluster)  [unwired: 4 in, 1 out]
            n278 = Flush File(refnum=w326, error in=w327) -> (refnum out=w325:refnum<file>, error out=w324:errorcluster)
            n279 = Close File(refnum=w325, error in=w324) -> ()  [unwired: 2 out]
          }
        }
      }
      event "运行间隔": Mouse Down {
        n280 = event-data() -> ("CtlRef"=w339:refnum<vi>)  [unwired: 1 in, 7 out]
        n281 = property class="DigNum (严格)"(reference=w339) -> (reference out=w338:refnum<vi>, "Value"=w337:i16)  [unwired: 1 in, 1 out]
        n282 = call "数字键盘.vi"("OldNumber"=w337) -> ("NewNumber"=w336:sgl)
        n283 = property class="DigNum (严格)"(reference=w338, "Val(Sgnl)"=w336) -> ()  [unwired: 1 in, 2 out]
      }
      event "流量阈值": Mouse Down {
        n284 = event-data() -> ("CtlRef"=w343:refnum<vi>)  [unwired: 1 in, 7 out]
        n285 = property class="DigNum (严格)"(reference=w343) -> (reference out=w342:refnum<vi>, "Value"=w341:dbl)  [unwired: 1 in, 1 out]
        n286 = call "数字键盘.vi"("OldNumber"=w341) -> ("NewNumber"=w340:sgl)
        n287 = property class="DigNum (严格)"(reference=w342, "Val(Sgnl)"=w340) -> ()  [unwired: 1 in, 2 out]
      }
      event "时间阈值": Mouse Down {
        n288 = event-data() -> ("CtlRef"=w347:refnum<vi>)  [unwired: 1 in, 7 out]
        n289 = property class="DigNum (严格)"(reference=w347) -> (reference out=w346:refnum<vi>, "Value"=w345:u16)  [unwired: 1 in, 1 out]
        n290 = call "数字键盘.vi"("OldNumber"=w345) -> ("NewNumber"=w344:sgl)
        n291 = property class="DigNum (严格)"(reference=w346, "Val(Sgnl)"=w344) -> ()  [unwired: 1 in, 2 out]
      }
      event "开机启动": Value Change {
        n292 = event-data() -> ("NewVal"=w349:bool)  [unwired: 1 in, 5 out]
        n293 = call <vilib>:"Application Directory.vi"() -> ("Application Directory"=w348:path)
        n294 = case shown="真" w349 {
          tunnel: w348 -> [w351 w355]
          frame False {
            n295 = call "删除启动项.vi"("启动文件路径"=w351) -> ("删除标记"=w350:bool)  [unwired: 9 in, 1 out]
            n296 = case shown="真" w350 {
              frame False {
                n297 = local write "开机启动"(TRUE ("开机启动")) -> ()
                n298 = One Button Dialog(message="启动项删除失败" ("消息")) -> ()  [unwired: 1 in, 1 out]
              }
              frame True {
              }
            }
          }
          frame True {
            n299 = call "添加启动项.vi"("启动文件路径"=w355) -> ("添加成功标记"=w354:bool)  [unwired: 9 in, 1 out]
            n300 = case shown="真" w354 {
              frame False {
                n301 = local write "开机启动"(FALSE ("开机启动")) -> ()
                n302 = One Button Dialog(message="启动项添加失败" ("消息")) -> ()  [unwired: 1 in, 1 out]
              }
              frame True {
              }
            }
          }
        }
      }
      event "副屏显示设置": Value Change {
        n303 = event-data() -> ()  [unwired: 1 in, 6 out]
        n304 = call "副屏设置.vi"() -> ()  [unwired: 12 in]
      }
      event "首页显示设置": Value Change {
        n305 = event-data() -> ()  [unwired: 1 in, 6 out]
        n306 = call "首页显示设置.vi"() -> ()  [unwired: 12 in]
      }
      event "短信报警设置": Value Change {
        n307 = event-data() -> ()  [unwired: 1 in, 6 out]
        n308 = invoke class="VI" method="FP.Open"(reference=w360, "Activate"=TRUE ("激活？"), "State"=T5."Standard" ("状态")) -> ()  [unwired: 2 in, 5 out]
      }
      event "布尔": Value Change {
        n309 = event-data() -> ("OldVal"=w362:bool)  [unwired: 1 in, 5 out]
        n310 = case shown="假" w362 {
          tunnel: [w363 _] -> w361
          frame False {
            n311 = call "数字密码键盘.vi"() -> ("NewNumber"=w363:sgl)  [unwired: 1 in]
          }
          frame True {
          }
        }
        n312 = local write "输入密码"(w361) -> ()
      }
    }
  }
